vi "UIM Programmatic User Modes.vi"() -> ()   [LabVIEW 2015]
doc: "This examples shows how you can programmatically capture UIM state, by iterating through all control properties in the start of the application, capturing them and then programatically selecting which mode should be applied."
uses:
  UIM/UIM.lvclass
panel:
  in  "Lock UI":bool
  in  "Remove Test":bool
  in  "Add Test":bool
  in  "Operator Information":bool
  in  "Configure Advanced":bool
  in  "Run Test":bool
  in  "Stop Button":bool
  in  "UI State":u16(ring) items=["Operator", "Admin"]
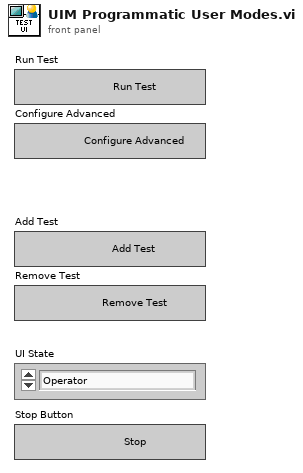
[diagram p1: front panel]
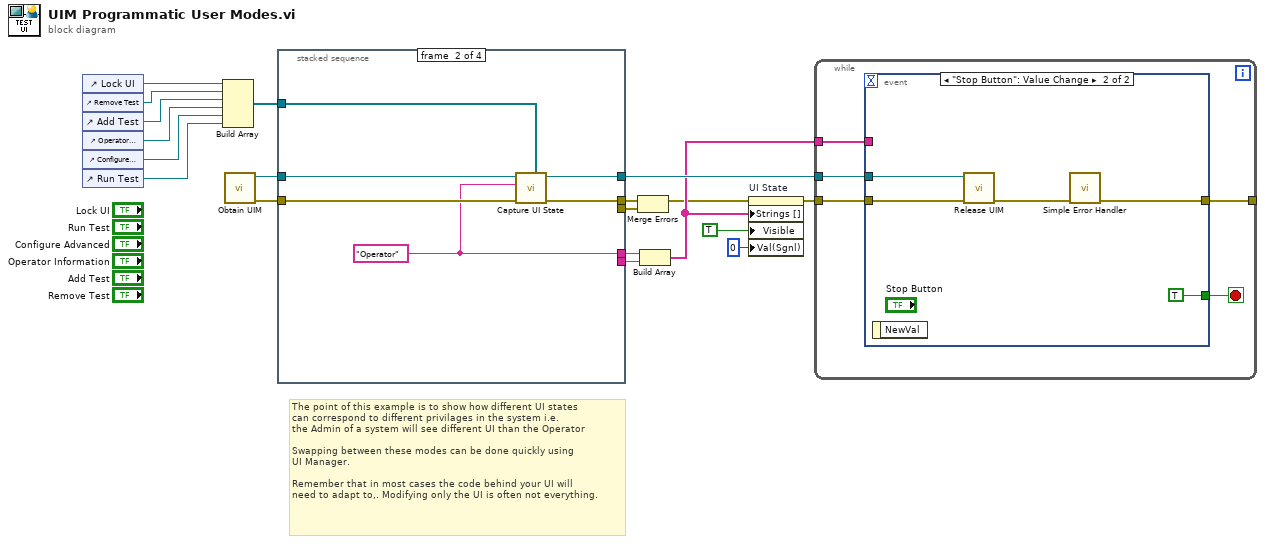
[diagram p0: block diagram]
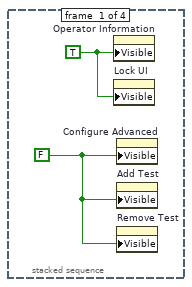
[diagram p2: hidden frame]
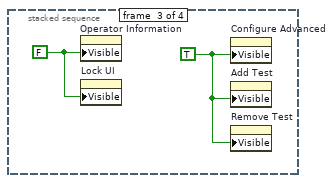
[diagram p3: hidden frame]
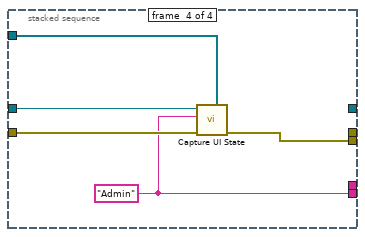
[diagram p4: hidden frame]
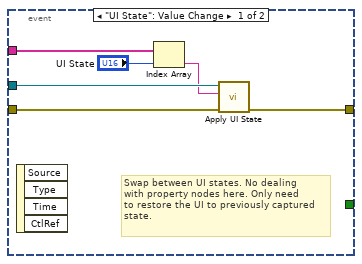
[diagram p5: hidden frame]
diagram:
  # "The point of this example is to show how different UI states\ncan correspond to different privilages in the system i.e.\nthe Admin of a system will see different UI than the Operator\n\nSwapping between these modes can be done quickly using\nUI Manager. \n\nRemember that in most cases the code behind your UI will\nneed to adapt to,. Modifying only the UI is often not everything."
  n1 = control-ref of="Lock UI"() -> (w11:refnum<vi>)
  n2 = control-ref of="Remove Test"() -> (w10:refnum<vi>)
  n3 = control-ref of="Add Test"() -> (w9:refnum<vi>)
  n4 = control-ref of="Operator Information"() -> (w8:refnum<vi>)
  n5 = control-ref of="Configure Advanced"() -> (w7:refnum<vi>)
  n6 = control-ref of="Run Test"() -> (w6:refnum<vi>)
  n7 = Build Array(w11, w10, w9, w8, w7, w6) -> (w5:refnum<vi>[])
  n8 = call "Obtain UIM.vi"() -> ("Error Out"=w15:errorcluster, "UIM Handle"=w16:refnum<data-value>)  [unwired: 10 in]
  n9 = stacked-sequence {
    tunnel: [_ w26 _ _] -> w17
    tunnel: w16 -> [_ w27 _ w34]
    tunnel: w15 -> [_ w25 _ w33]
    tunnel: [_ w24 _ _] -> w14
    tunnel: [_ w23 _ _] -> w13
    tunnel: w5 -> [_ w22 _ w31]
    tunnel: [_ _ _ w32] -> w3
    tunnel: [_ _ _ w30] -> w2
    frame #0 {
      w20 = TRUE
      w21 = FALSE
      n10 = property on="Operator Information" class="Bool"("Visible"=w20) -> ()  [unwired: 2 in, 2 out]
      n11 = property on="Lock UI" class="Bool"("Visible"=w20) -> ()  [unwired: 2 in, 2 out]
      n12 = property on="Configure Advanced" class="Bool"("Visible"=w21) -> ()  [unwired: 2 in, 2 out]
      n13 = property on="Add Test" class="Bool"("Visible"=w21) -> ()  [unwired: 2 in, 2 out]
      n14 = property on="Remove Test" class="Bool"("Visible"=w21) -> ()  [unwired: 2 in, 2 out]
    }
    frame #1 {
      w23 = "Operator" ("State Name")
      n15 = call "Capture UI State.vi"("Ctls Refs (All Ctls)"=w22, "Error In"=w25, "State Name"=w23, "UIM In"=w27) -> ("Error Out"=w24:errorcluster, "UIM Out"=w26:refnum<data-value>)  [unwired: 6 in]
    }
    frame #2 {
      w28 = FALSE
      w29 = TRUE
      n16 = property on="Operator Information" class="Bool"("Visible"=w28) -> ()  [unwired: 2 in, 2 out]
      n17 = property on="Lock UI" class="Bool"("Visible"=w28) -> ()  [unwired: 2 in, 2 out]
      n18 = property on="Configure Advanced" class="Bool"("Visible"=w29) -> ()  [unwired: 2 in, 2 out]
      n19 = property on="Add Test" class="Bool"("Visible"=w29) -> ()  [unwired: 2 in, 2 out]
      n20 = property on="Remove Test" class="Bool"("Visible"=w29) -> ()  [unwired: 2 in, 2 out]
    }
    frame #3 {
      w30 = "Admin" ("State Name")
      n21 = call "Capture UI State.vi"("Ctls Refs (All Ctls)"=w31, "Error In"=w33, "State Name"=w30, "UIM In"=w34) -> ("Error Out"=w32:errorcluster)  [unwired: 6 in, 1 out]
    }
  }
  n22 = Merge Errors(w14, w3) -> (w4:errorcluster)
  n23 = Build Array(w13, w2) -> (w12:string[])
  n24 = property on="UI State" class="Ring (strict)"(error in=w4, "Strings []"=w12, "Visible"=TRUE, "Val(Sgnl)"=u16 0 ("Value (Signaling)")) -> (error out=w19:errorcluster)  [unwired: 1 in, 1 out]
  n25 = while {
    tunnel: w17 -> [w39]
    tunnel: w19 -> [w37]
    tunnel: [w36] -> _
    tunnel: w12 -> [w35]
    stop <- w38 stop-if-true
    n26 = event shown="[1] \"Stop Button\": Value Change" {
      selector: _ -> [_ _]
      dyn-events: _ -> [_ _]
      timeout: _ -> [_ _]
      tunnel: w39 -> [w45 w49]
      tunnel: [_ TRUE] -> w38
      tunnel: w37 -> [w44 w48]
      tunnel: [w43 w46] -> w36
      tunnel: w35 -> [w40 _]
      event "UI State": Value Change {
        # "Swap between UI states. No dealing\nwith property nodes here. Only need\nto restore the UI to previously captured\nstate."
        n27 = event-data() -> ()  [unwired: 1 in, 4 out]
        n28 = Index Array(array=w40, index="UI State") -> (element=w41:string)
        n29 = call "Apply UI State.vi"("Error In"=w44, "State Name"=w41, "UIM In"=w45) -> ("Error Out"=w43:errorcluster)  [unwired: 7 in, 1 out]
      }
      event "Stop Button": Value Change {
        n30 = event-data() -> ()  [unwired: 1 in, 1 out]
        n31 = call "Release UIM.vi"("Error In"=w48, "UIM Handle"=w49) -> ("Error Out"=w47:errorcluster)  [unwired: 9 in]
        n32 = call <vilib>:"Simple Error Handler.vi"("error in (no error)"=w47) -> ("error out"=w46:errorcluster)  [unwired: 4 in, 4 out]
      }
    }
  }
